vi "DriveAzimuthOutput.vi"() -> ()   [LabVIEW 2019]
uses:
  <vilib>/Rock Robotics/WPI/ThirdParty/REV Robotics/SPARK MAX/Typedef/Spark MAX Idle Mode.ctl
  b0ab5e4e-5e25-4fd8-81a8-60ad2610010b.vi
  0974dfea-b596-4a4a-8f8a-14ad5d990518.vi
  a584ed06-9e0e-4cf2-9e41-46fb601cb602.vi
  fae3915a-5fd6-4bed-a8f4-656c81b67242.vi
  refnums.vi
  GRNF_GenericMotor.vi
  outputs.vi
  sensors.vi
panel:
  out "Controller Summary":T1(graph)
  in  "PID Tuning Parameters":T2={"Kp"=0.005, "Ki"=0.0, "Kd"=0.0, "N-Diff"=10, "N-Int"=10, "Int Error Window"=180.0, "Max Ouput"=1.0, "Min Output"=-1.0} {"Int Error Window" min=0.0; "N-Int" min=2; "N-Diff" min=2; "Kd" min=0.0; "Ki" min=0.0; "Kp" min=0.0}
  in  "Plot Azimuth":bool
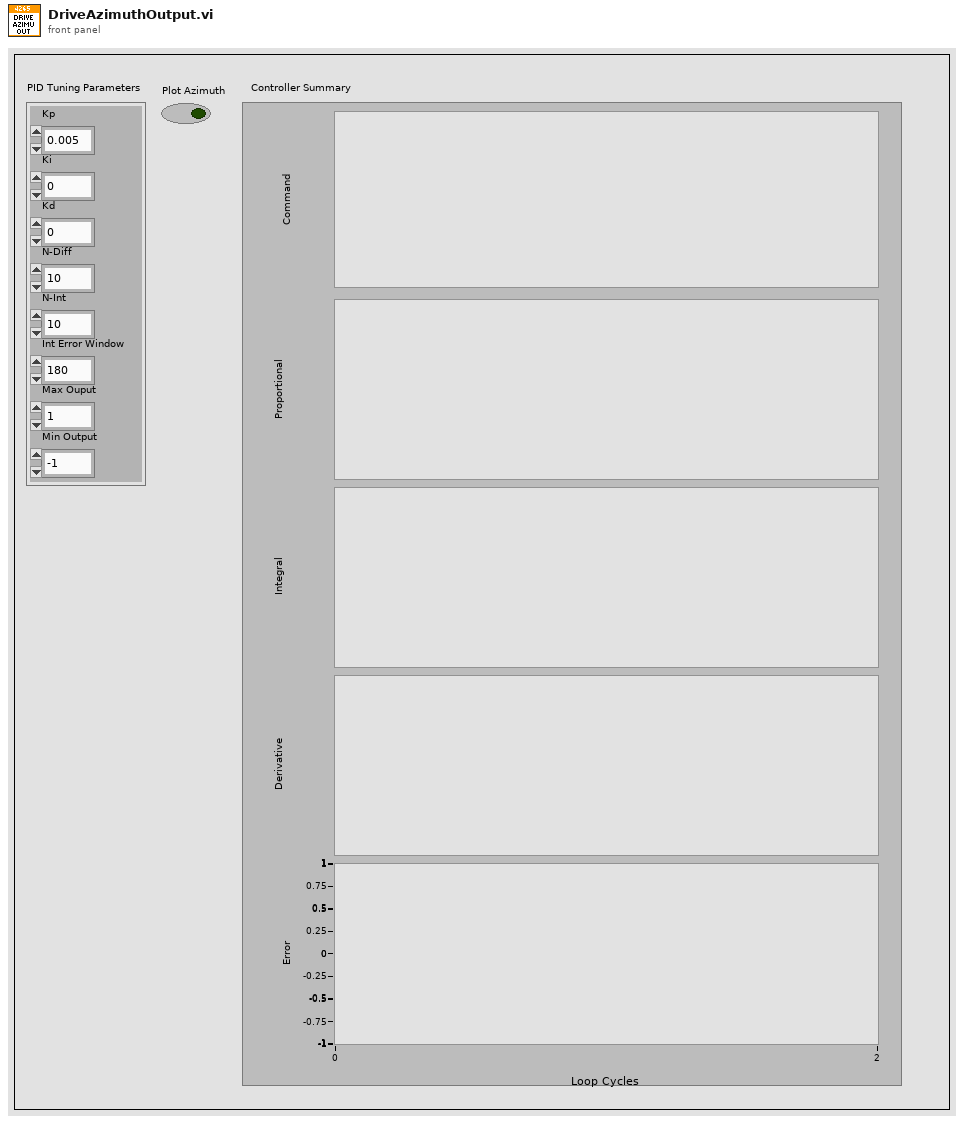
[diagram p1: front panel]
types:
  T1 = cluster{"Command":dbl, "Proportional":dbl, "Integral":dbl, "Derivative":dbl, "Goal":dbl}
  T2 = cluster{"Kp":dbl, "Ki":dbl, "Kd":dbl, "N-Diff":i32, "N-Int":i32, "Int Error Window":dbl, "Max Ouput":dbl, "Min Output":dbl}
  T3 = typedef "WPI_MotorControlDeviceRef.ctl" = cluster{"DeviceStatus":errorcluster, "Type":T4, "PWM":cluster{"PWM Channel":T5, "DeadBand":T6}, "CAN":cluster{"Device Number":u8, "SetOutput VI Ref":variant, "GetOutput VI Ref":variant, "Enable VI Ref":variant, "Disable VI Ref":variant, "Data":variant}, "Invert":bool, "DIO PWM":cluster{"PWM \"Enable\" Channel":T5, "DIOChannel":T7, "PWM Rate":dbl}}
  T4 = typedef "WPI_MotorControlType.ctl" = enum16{"PWM", "CAN", "DIO PWM"}
  T5 = typedef "FPGA_DIOPWMChannel.ctl" = enum8{"PWM 0", "PWM 1", "PWM 2", "PWM 3", "PWM 4", "PWM 5", "PWM 6", "PWM 7", "PWM 8", "PWM 9", "PWM MXP 0", "PWM MXP 1", "PWM MXP 2", "PWM MXP 3", "PWM MXP 4", "PWM MXP 5", "PWM MXP 6", "PWM MXP 7", "PWM MXP 8", "PWM MXP 9", "Invalid"}
  T6 = typedef "WPI_PWMDeadband.ctl" = cluster{"Name":string, "maxPositivePwm":i32, "minPositivePwm":i32, "centerPwm":i32, "maxNegativePwm":i32, "minNegativePwm":i32, "angularRange":u16}
  T7 = typedef "FPGA_DIOChannel.ctl" = enum8{"DIO 0", "DIO 1", "DIO 2", "DIO 3", "DIO 4", "DIO 5", "DIO 6", "DIO 7", "DIO 8", "DIO 9", "DIO MXP 0", "DIO MXP 1", "DIO MXP 2", "DIO MXP 3", "DIO MXP 4", "DIO MXP 5", "DIO MXP 6", "DIO MXP 7", "DIO MXP 8", "DIO MXP 9", "DIO MXP 10", "DIO MXP 11", "DIO MXP 12", "DIO MXP 13", "DIO MXP 14", "DIO MXP 15", "SPI Port CS1", "SPI Port CS2", "SPI Port CS3", "SPI Port MISO", "SPI Port MOSI", "Invalid"}
  T8 = typedef "Spark MAX Idle Mode.ctl" = enum16{"Coast", "Brake"}
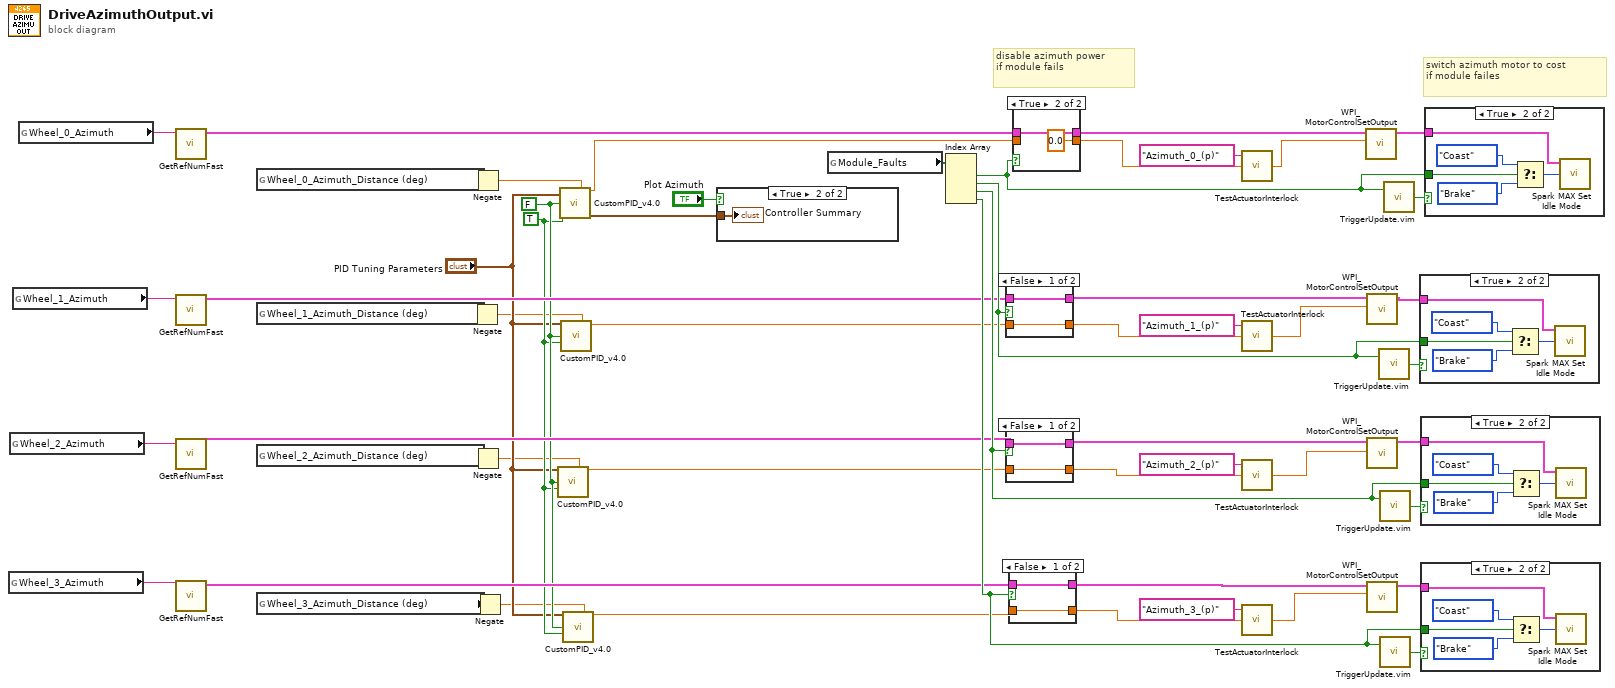
[diagram p0: block diagram]
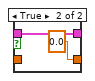
[diagram p6: hidden frame]
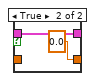
[diagram p7: hidden frame]
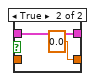
[diagram p8: hidden frame]
diagram:
  w9 = FALSE ("Reset on Goal Change ?")
  w8 = TRUE ("Use Custom Error Calculation ?")
  # "switch azimuth motor to cost\nif module failes"
  # "disable azimuth power\nif module fails"
  n1 = global read "refnums.vi" "Wheel_3_Azimuth"() -> (w17:string)
  n2 = global read "refnums.vi" "Wheel_2_Azimuth"() -> (w18:string)
  n3 = global read "refnums.vi" "Wheel_1_Azimuth"() -> (w19:string)
  n4 = global read "refnums.vi" "Wheel_0_Azimuth"() -> (w20:string)
  n5 = call-poly "GetRefNumFast.vi"("RefNum Name"=w20) -> ("Device Reference"=w24:T3)  [unwired: 5 in, 1 out]
  n6 = call-poly "GetRefNumFast.vi"("RefNum Name"=w19) -> ("Device Reference"=w23:T3)  [unwired: 5 in, 1 out]
  n7 = call-poly "GetRefNumFast.vi"("RefNum Name"=w18) -> ("Device Reference"=w22:T3)  [unwired: 5 in, 1 out]
  n8 = call-poly "GetRefNumFast.vi"("RefNum Name"=w17) -> ("Device Reference"=w21:T3)  [unwired: 5 in, 1 out]
  n9 = global read "outputs.vi" "Wheel_0_Azimuth_Distance (deg)"() -> (w16:dbl)
  n10 = global read "outputs.vi" "Wheel_1_Azimuth_Distance (deg)"() -> (w13:dbl)
  n11 = global read "outputs.vi" "Wheel_2_Azimuth_Distance (deg)"() -> (w11:dbl)
  n12 = global read "outputs.vi" "Wheel_3_Azimuth_Distance (deg)"() -> (w10:dbl)
  n13 = Negate(x=w13) -> (-x=w3:dbl)
  n14 = Negate(x=w16) -> (-x=w4:dbl)
  n15 = Negate(x=w11) -> (-x=w2:dbl)
  n16 = Negate(x=w10) -> (-x=w1:dbl)
  n17 = call "CustomPID_v4.0.vi"("PID Tuning Parameters"="PID Tuning Parameters", "Custom Error Calculation"=w2, "Reset on Goal Change ?"=w9, "Use Custom Error Calculation ?"=w8) -> ("Command"=w5:dbl)  [unwired: 8 in, 3 out]
  n18 = call "CustomPID_v4.0.vi"("PID Tuning Parameters"="PID Tuning Parameters", "Custom Error Calculation"=w4, "Reset on Goal Change ?"=w9, "Use Custom Error Calculation ?"=w8) -> ("Command"=w15:dbl, "Controller Summary"=w14:T1)  [unwired: 8 in, 2 out]
  n19 = call "CustomPID_v4.0.vi"("PID Tuning Parameters"="PID Tuning Parameters", "Custom Error Calculation"=w3, "Reset on Goal Change ?"=w9, "Use Custom Error Calculation ?"=w8) -> ("Command"=w12:dbl)  [unwired: 8 in, 3 out]
  n20 = call "CustomPID_v4.0.vi"("PID Tuning Parameters"="PID Tuning Parameters", "Custom Error Calculation"=w1, "Reset on Goal Change ?"=w9, "Use Custom Error Calculation ?"=w8) -> ("Command"=w6:dbl)  [unwired: 8 in, 3 out]
  n21 = case shown="True" "Plot Azimuth" {
    tunnel: w14 -> [_ w55]
    frame False {
    }
    frame True {
      "Controller Summary" <- w55
    }
  }
  n22 = global read "sensors.vi" "Module_Faults"() -> (w30:bool[])
  n23 = Index Array(array=w30) -> (element #1=w32:bool, element #2=w36:bool, element #3=w39:bool, element #4=w42:bool)  [unwired: 4 in]
  n24 = case shown="False" w36 {
    tunnel: [w57 w59] -> w27
    tunnel: w23 -> [w57 w59]
    tunnel: [w56 0.0 ("Command")] -> w47
    tunnel: w12 -> [w56 _]
    frame False {
    }
    frame True {
    }
  }
  n25 = case shown="False" w39 {
    tunnel: [w61 w63] -> w28
    tunnel: w22 -> [w61 w63]
    tunnel: [w60 0.0 ("Command")] -> w50
    tunnel: w5 -> [w60 _]
    frame False {
    }
    frame True {
    }
  }
  n26 = case shown="False" w42 {
    tunnel: [w65 w67] -> w29
    tunnel: w21 -> [w65 w67]
    tunnel: [w64 0.0 ("Command")] -> w53
    tunnel: w6 -> [w64 _]
    frame False {
    }
    frame True {
    }
  }
  n27 = case shown="True" w32 {
    tunnel: [w69 w71] -> w26
    tunnel: w24 -> [w69 w71]
    tunnel: [w68 0.0 ("Command")] -> w44
    tunnel: w15 -> [w68 _]
    frame False {
    }
    frame True {
    }
  }
  n28 = call "TestActuatorInterlock.vi"("Input_Value_Double"=w44, "Actuator_Name"="Azimuth_0_(p)") -> ("Output_Value_Double"=w45:dbl)  [unwired: 1 in, 2 out]
  n29 = call "TestActuatorInterlock.vi"("Input_Value_Double"=w47, "Actuator_Name"="Azimuth_1_(p)") -> ("Output_Value_Double"=w48:dbl)  [unwired: 1 in, 2 out]
  n30 = call "TestActuatorInterlock.vi"("Input_Value_Double"=w50, "Actuator_Name"="Azimuth_2_(p)") -> ("Output_Value_Double"=w51:dbl)  [unwired: 1 in, 2 out]
  n31 = call "TestActuatorInterlock.vi"("Input_Value_Double"=w53, "Actuator_Name"="Azimuth_3_(p)") -> ("Output_Value_Double"=w54:dbl)  [unwired: 1 in, 2 out]
  n32 = call <vilib>:"WPI_MotorControlSetOutput.vi"("Output"=w45, "MotorControlDevRef"=w26) -> ("MotorControlDevRef"=w33:T3)  [unwired: 7 in, 2 out]
  n33 = call <vilib>:"WPI_MotorControlSetOutput.vi"("Output"=w48, "MotorControlDevRef"=w27) -> ("MotorControlDevRef"=w35:T3)  [unwired: 7 in, 2 out]
  n34 = call <vilib>:"WPI_MotorControlSetOutput.vi"("Output"=w51, "MotorControlDevRef"=w28) -> ("MotorControlDevRef"=w38:T3)  [unwired: 7 in, 2 out]
  n35 = call <vilib>:"WPI_MotorControlSetOutput.vi"("Output"=w54, "MotorControlDevRef"=w29) -> ("MotorControlDevRef"=w41:T3)  [unwired: 7 in, 2 out]
  n36 = call "TriggerUpdate.vim"("Trigger"=w36) -> ("Update"=w34:bool)  [unwired: 1 in]
  n37 = call "TriggerUpdate.vim"("Trigger"=w39) -> ("Update"=w37:bool)  [unwired: 1 in]
  n38 = call "TriggerUpdate.vim"("Trigger"=w42) -> ("Update"=w40:bool)  [unwired: 1 in]
  n39 = call "TriggerUpdate.vim"("Trigger"=w32) -> ("Update"=w31:bool)  [unwired: 1 in]
  n40 = case shown="True" w34 {
    tunnel: w36 -> [_ w73]
    tunnel: w35 -> [_ w72]
    frame False {
    }
    frame True {
      n41 = Select(t=Spark_MAX_Idle_Mode."Coast" ("Idle Mode"), s=w73, f=Spark_MAX_Idle_Mode."Brake" ("Idle Mode")) -> (s? t:f=w74:T8)
      n42 = call <vilib>:"Spark MAX Set Idle Mode.vi"("Idle Mode"=w74, "MotorControlDeviceRef in"=w72) -> ()  [unwired: 8 in, 2 out]
    }
  }
  n43 = case shown="True" w37 {
    tunnel: w39 -> [_ w78]
    tunnel: w38 -> [_ w77]
    frame False {
    }
    frame True {
      n44 = Select(t=Spark_MAX_Idle_Mode."Coast" ("Idle Mode"), s=w78, f=Spark_MAX_Idle_Mode."Brake" ("Idle Mode")) -> (s? t:f=w79:T8)
      n45 = call <vilib>:"Spark MAX Set Idle Mode.vi"("Idle Mode"=w79, "MotorControlDeviceRef in"=w77) -> ()  [unwired: 8 in, 2 out]
    }
  }
  n46 = case shown="True" w40 {
    tunnel: w42 -> [_ w83]
    tunnel: w41 -> [_ w82]
    frame False {
    }
    frame True {
      n47 = Select(t=Spark_MAX_Idle_Mode."Coast" ("Idle Mode"), s=w83, f=Spark_MAX_Idle_Mode."Brake" ("Idle Mode")) -> (s? t:f=w84:T8)
      n48 = call <vilib>:"Spark MAX Set Idle Mode.vi"("Idle Mode"=w84, "MotorControlDeviceRef in"=w82) -> ()  [unwired: 8 in, 2 out]
    }
  }
  n49 = case shown="True" w31 {
    tunnel: w32 -> [_ w88]
    tunnel: w33 -> [_ w87]
    frame False {
    }
    frame True {
      n50 = Select(t=Spark_MAX_Idle_Mode."Coast" ("Idle Mode"), s=w88, f=Spark_MAX_Idle_Mode."Brake" ("Idle Mode")) -> (s? t:f=w89:T8)
      n51 = call <vilib>:"Spark MAX Set Idle Mode.vi"("Idle Mode"=w89, "MotorControlDeviceRef in"=w87) -> ()  [unwired: 8 in, 2 out]
    }
  }
